vi "Get_recomendation.vi"(7 "LabVIEW Web Service Request":refnum<class "Web Request.lvclass">, 10 "Part_param_json":string) -> (2 "Recommendation":string)   [LabVIEW 2020]
uses:
  <vilib>/wsapi/Web Request.lvclass
  <vilib>/Utility/error.llb/DialogType.ctl
  <vilib>/addons/database/Connection.llb/DB Tools Open Connec (Path).vi
  <vilib>/addons/database/NI_Database_API.lvlib
panel:
  out "data":string[][](array[string])
  out "Part_param":T1
  # "Use the Web Service Request input terminal to call the VIs on the Web Services palette. Do not remove it from the connector pane unless you don't need access to the palette."
  # "Each additional control wired to the connector pane will be available as an input in the URL. To include an indicator in terminal-mode output (the default setting), it must also be wired to the connector pane."
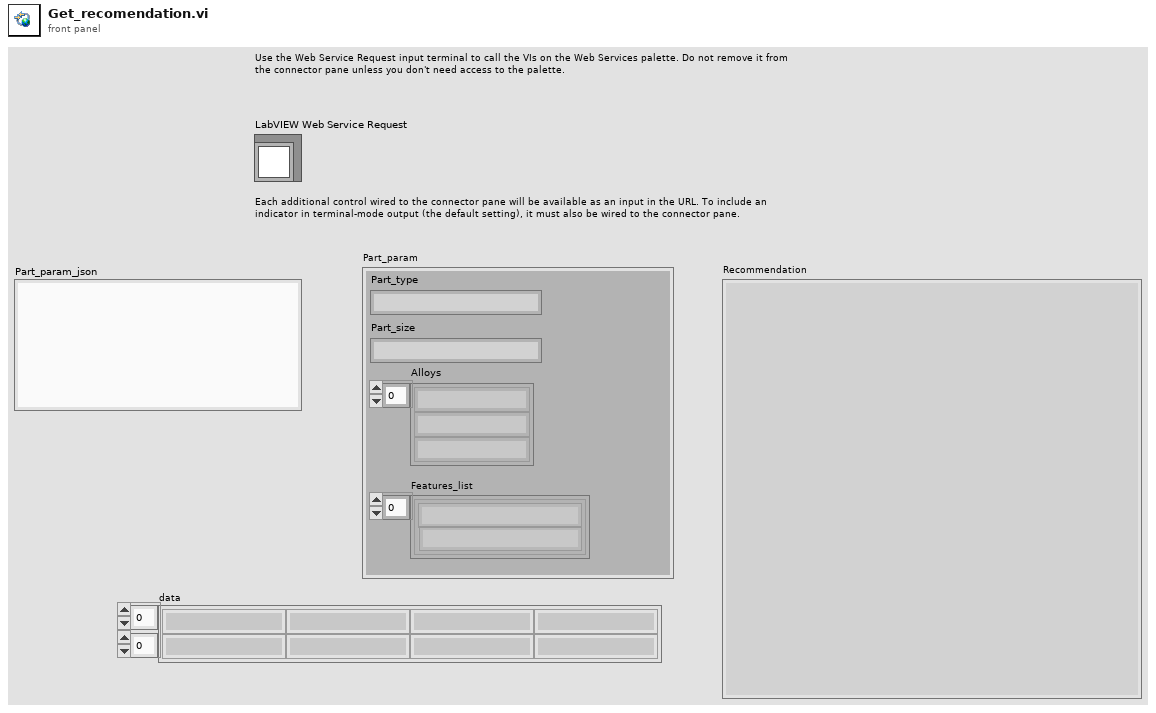
[diagram p1: front panel]
types:
  T1 = cluster{"Part_type":string, "Part_size":string, "Alloys":string[], "Features_list":cluster{"Feature_name":string, "Value":string}[]}
  T2 = cluster{"Electolyte_Name":string, "Electolyte_Formula":string, "Mode_name":string, "Process_Duration":string, "Additional_Operation":string}
  T3 = typedef "NI_Database_API.lvlib/Conn ObjectReference.ctl" = refnum<k1>
  T4 = typedef "DialogType.ctl" = u16
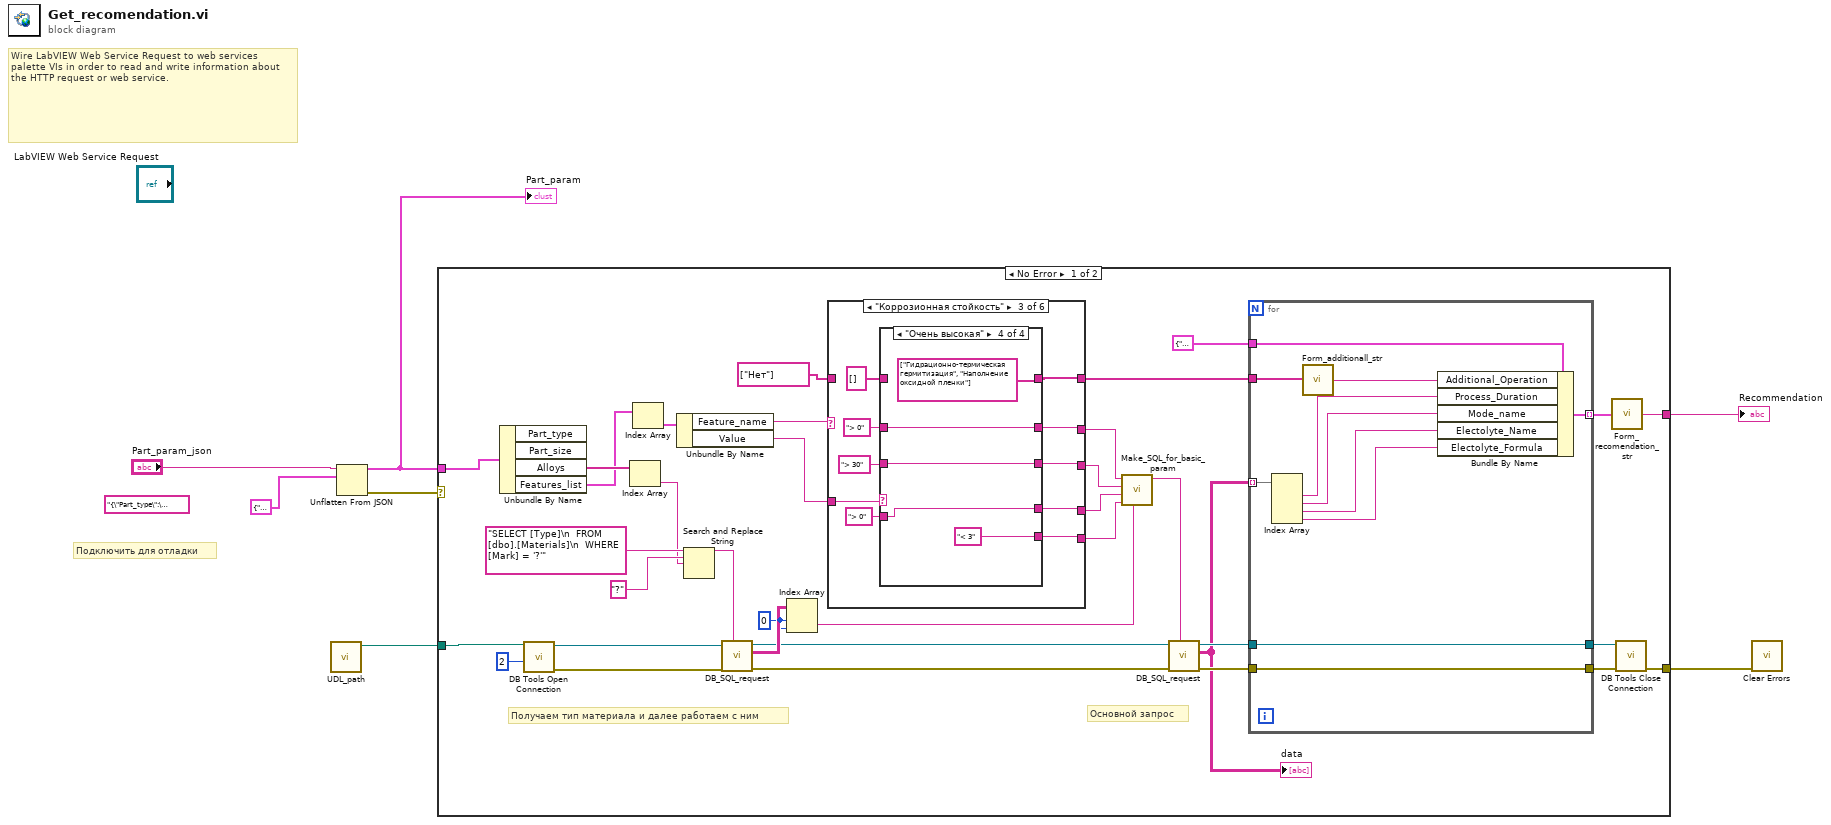
[diagram p0: block diagram]
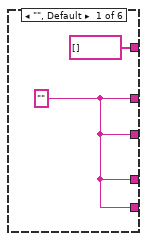
[diagram p2: hidden frame]
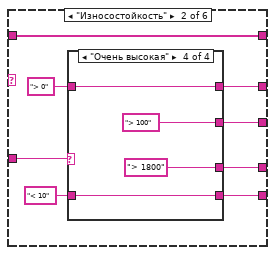
[diagram p3: hidden frame]
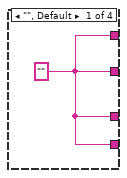
[diagram p4: hidden frame]
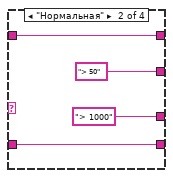
[diagram p5: hidden frame]
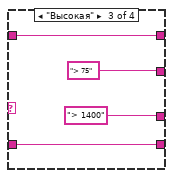
[diagram p6: hidden frame]
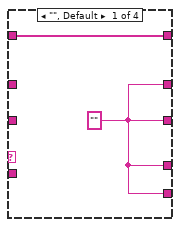
[diagram p7: hidden frame]
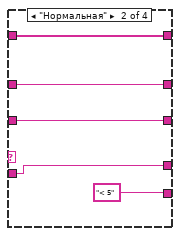
[diagram p8: hidden frame]
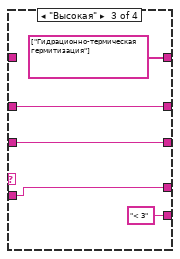
[diagram p9: hidden frame]
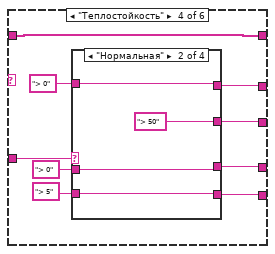
[diagram p10: hidden frame]
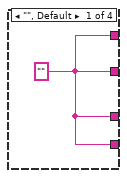
[diagram p11: hidden frame]
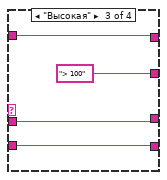
[diagram p12: hidden frame]
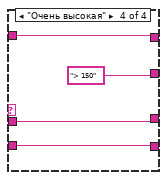
[diagram p13: hidden frame]
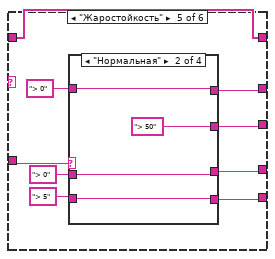
[diagram p14: hidden frame]
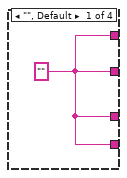
[diagram p15: hidden frame]
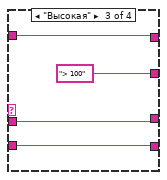
[diagram p16: hidden frame]
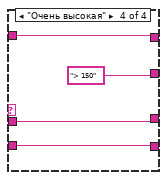
[diagram p17: hidden frame]
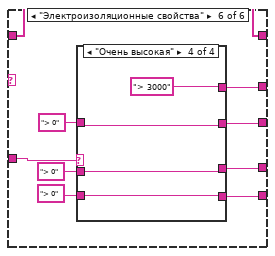
[diagram p18: hidden frame]
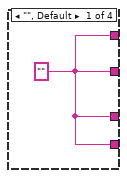
[diagram p19: hidden frame]
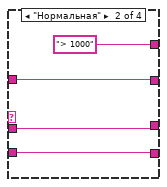
[diagram p20: hidden frame]
diagram:
  (unwired) "{\"Part_type\":\"Пластина\",\"Part_size\":\"0,05-0,1 дм2\",\"Alloys\":[\"АД000\"],\"Features_list\":[{\"Feature_name\":\"Износостойкость\",\"Value\":\"Нормальная\"}]}" ("Part_param_json")
  # "Подключить для отладки"
  # "Wire LabVIEW Web Service Request to web services palette VIs in order to read and write information about the HTTP request or web service."
  n1 = call "UDL_path.vi"() -> ("Path"=w6:path)  [unwired: 11 in]
  n2 = Unflatten From JSON(JSON string="Part_param_json", type and defaults=T1 {"Part_type"="", "Part_size"="", "Alloys"=[], "Features_list"=[]} ("Part_param")) -> (value=w1:T1, error out=w4:errorcluster)  [unwired: 5 in]
  "Part_param" <- w1
  n3 = case shown="No Error" w4 {
    selector: w4 -> [_ w170]
    tunnel: w1 -> [w42 _]
    tunnel: w6 -> [w39 _]
    tunnel: [w36 w170] -> w3
    tunnel: [w14 w171] -> w5
    frame No Error {
      w31 = 0 ("index (row)")
      # "Основной запрос"
      # "Получаем тип материала и далее работаем с ним"
      n4 = Unbundle By Name(w42) -> ("Alloys"=w41:string[], "Features_list"=w11:cluster{"Feature_name":string, "Value":string}[])  [unwired: 2 out]
      n5 = call-poly <vilib>:"DB Tools Open Connection.vi"("connection timeout (15)"=2, "connection information"=w39) -> ("error out"=w38:errorcluster, "connection reference"=w37:T3)  [unwired: 6 in]
      n6 = Index Array(array=w41) -> (element=w12:string)  [unwired: 1 in]
      n7 = Index Array(array=w11) -> (element=w10:cluster{"Feature_name":string, "Value":string})  [unwired: 1 in]
      n8 = Unbundle By Name(w10) -> ("Feature_name"=w9:string, "Value"=w8:string)
      n9 = Search and Replace String(input string="SELECT [Type]\n  FROM [dbo].[Materials]\n  WHERE [Mark] = '?'" ("SQL query"), search string="?", replace string=w12) -> (result string=w34:string)  [unwired: 5 in, 3 out]
      n10 = call "DB_SQL_request.vi"("SQL query"=w34, "error in (no error)"=w38, "Refnum in"=w37) -> ("error out"=w29:errorcluster, "data"=w32:string[][], "Refnum out"=w28:T3)  [unwired: 6 in]
      n11 = Index Array(array=w32, index (row)=w31, index (col)=w31) -> (element=w30:string)
      n12 = case shown="\"Коррозионная стойкость\"" w9 {
        tunnel: w8 -> [_ w63 w86 w112 w131 w154]
        tunnel: [w55 w59 w81 w110 w130 w153] -> w26
        tunnel: [w55 w62 w85 w109 w129 w149] -> w25
        tunnel: [w55 w61 w84 w106 w128 w150] -> w24
        tunnel: [w55 w57 w83 w107 w127 w151] -> w23
        tunnel: [string[] [] w56 w78 w104 w126 w148] -> w17
        tunnel: string[] ["Нет"] -> [_ w56 _ w104 w126 w148]
        frame "", Default {
          w55 = ""
        }
        frame "Износостойкость" {
          n13 = case shown="\"Очень высокая\"" w63 {
            tunnel: [w64 w67 w71 w75] -> w59
            tunnel: [w64 "> 50" "> 75" "> 100"] -> w62
            tunnel: [w64 "> 1000" "> 1400" "> 1800"] -> w61
            tunnel: [w64 w66 w72 w76] -> w57
            tunnel: "> 0" -> [_ w67 w71 w75]
            tunnel: "< 10" -> [_ w66 w72 w76]
            frame "", Default {
              w64 = ""
            }
            frame "Нормальная" {
            }
            frame "Высокая" {
            }
            frame "Очень высокая" {
            }
          }
        }
        frame "Коррозионная стойкость" {
          n14 = case shown="\"Очень высокая\"" w86 {
            tunnel: [w88 w92 w96 w101] -> w81
            tunnel: [w88 w91 w97 w102] -> w85
            tunnel: [w88 w90 w98 w103] -> w84
            tunnel: [w88 "< 5" "< 3" "< 3"] -> w83
            tunnel: "> 0" -> [_ w92 w96 w101]
            tunnel: "> 30" -> [_ w91 w97 w102]
            tunnel: "> 0" -> [_ w90 w98 w103]
            tunnel: [w87 w89 string[] ["Гидрационно-термическая гермитизация"] string[] ["Гидрационно-термическая гермитизация", "Наполнение оксидной пленки"]] -> w78
            tunnel: string[] [] -> [w87 w89 _ _]
            frame "", Default {
              w88 = ""
            }
            frame "Нормальная" {
            }
            frame "Высокая" {
            }
            frame "Очень высокая" {
            }
          }
        }
        frame "Теплостойкость" {
          n15 = case shown="\"Нормальная\"" w112 {
            tunnel: [w113 w117 w118 w124] -> w110
            tunnel: [w113 "> 50" "> 100" "> 150"] -> w109
            tunnel: [w113 w115 w120 w123] -> w106
            tunnel: [w113 w116 w119 w122] -> w107
            tunnel: "> 0" -> [_ w117 w118 w124]
            tunnel: "> 5" -> [_ w116 w119 w122]
            tunnel: "> 0" -> [_ w115 w120 w123]
            frame "", Default {
              w113 = ""
            }
            frame "Нормальная" {
            }
            frame "Высокая" {
            }
            frame "Очень высокая" {
            }
          }
        }
        frame "Жаростойкость" {
          n16 = case shown="\"Нормальная\"" w131 {
            tunnel: [w135 w139 w140 w146] -> w130
            tunnel: [w135 "> 50" "> 100" "> 150"] -> w129
            tunnel: [w135 w137 w142 w145] -> w128
            tunnel: [w135 w138 w141 w144] -> w127
            tunnel: "> 0" -> [_ w139 w140 w146]
            tunnel: "> 5" -> [_ w138 w141 w144]
            tunnel: "> 0" -> [_ w137 w142 w145]
            frame "", Default {
              w135 = ""
            }
            frame "Нормальная" {
            }
            frame "Высокая" {
            }
            frame "Очень высокая" {
            }
          }
        }
        frame "Электроизоляционные свойства" {
          n17 = case shown="\"Очень высокая\"" w154 {
            tunnel: [w157 "> 1000" "> 2000" "> 3000"] -> w153
            tunnel: [w157 w158 w163 w167] -> w149
            tunnel: [w157 w160 w165 w169] -> w150
            tunnel: [w157 w161 w164 w168] -> w151
            tunnel: "> 0" -> [_ w161 w164 w168]
            tunnel: "> 0" -> [_ w160 w165 w169]
            tunnel: "> 0" -> [_ w158 w163 w167]
            frame "", Default {
              w157 = ""
            }
            frame "Нормальная" {
            }
            frame "Высокая" {
            }
            frame "Очень высокая" {
            }
          }
        }
      }
      n18 = call "Make_SQL_for_basic_param.vi"("Material Type"=w30, "Porosity, %"=w23, "Hardness HV, kg/mm2"=w24, "Thickness, um"=w25, "Breakdown DC voltage, V"=w26) -> ("result string"=w27:string)  [unwired: 6 in]
      n19 = call "DB_SQL_request.vi"("SQL query"=w27, "error in (no error)"=w29, "Refnum in"=w28) -> ("error out"=w20:errorcluster, "data"=w19:string[][], "Refnum out"=w21:T3)  [unwired: 6 in]
      "data" <- w19
      n20 = for {
        tunnel: w21 -> [w48]
        tunnel: w20 -> [w49]
        tunnel: w19 -> [w52] mode=indexing
        tunnel: T2 {"Electolyte_Name"="", "Electolyte_Formula"="", "Mode_name"="", "Process_Duration"="", "Additional_Operation"=""} ("Recomendation") -> [w53]
        tunnel: w17 -> [w47]
        tunnel: [w50] -> w13 mode=indexing
        tunnel: [w49] -> w16
        tunnel: [w48] -> w15
        n21 = Index Array(array=w52) -> (element #1=w51:string, element #2=w45:string, element #3=w44:string, element #4=w43:string)  [unwired: 4 in]
        n22 = call "Form_additionall_str.vi"("Array"=w47) -> ("String"=w46:string)
        n23 = Bundle By Name(cluster=w53, "Additional_Operation"=w46, "Process_Duration"=w51, "Mode_name"=w45, "Electolyte_Name"=w44, "Electolyte_Formula"=w43) -> (w50:T2)
      }
      n24 = call "Form_recomendation_str.vi"("Recomendation_arr"=w13) -> ("Recomendation_str"=w14:string)
      n25 = call <vilib>:"DB Tools Close Connection.vi"("error in (no error)"=w16, "connection reference"=w15) -> ("error out"=w36:errorcluster)  [unwired: 5 in]
    }
    frame Error {
      w172 = T4 0 items=["no dialog", "OK message", "continue or stop message", "OK message + warnings", "continue/stop + warnings"] ("type of dialog (OK msg:1)")
      n26 = call <vilib>:"Simple Error Handler.vi"("type of dialog (OK msg:1)"=w172, "error in (no error)"=w170) -> ("message"=w171:string)  [unwired: 3 in, 4 out]
    }
  }
  "Recommendation" <- w5
  n27 = call <vilib>:"Clear Errors.vi"("error in (no error)"=w3) -> ()  [unwired: 5 in, 2 out]
